vi "test Get Attribute as JSON.vi"(11 "Test Case In":refnum<class "Test Config From EXCEL.lvclass">) -> (0 "error out":errorcluster, 3 "Test Case Out":refnum<class "Test Config From EXCEL.lvclass">)   [LabVIEW 2020, in "Test Config From EXCEL.lvclass"]
uses:
  Test Config From EXCEL.lvclass
  Test Config From EXCEL.lvclass/Test Config From EXCEL.ctl
  <vilib>/JDP Science/JSONtext/JSONtext.lvlib
  <vilib>/Astemes/LUnit/Test Case.lvclass
  <vilib>/Peter/Open Xml/Source/Open Xml.lvlib
  Source/Config from EXCEL/Config from EXCEL.lvclass
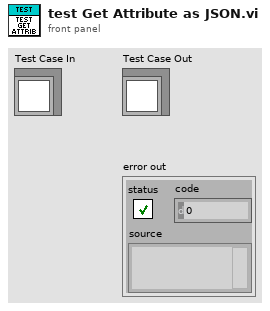
[diagram p1: front panel]
types:
  T1 = cluster{"Sheet Name":string, "Name":string, "Display Name":string, "Range or Cell Address":string}
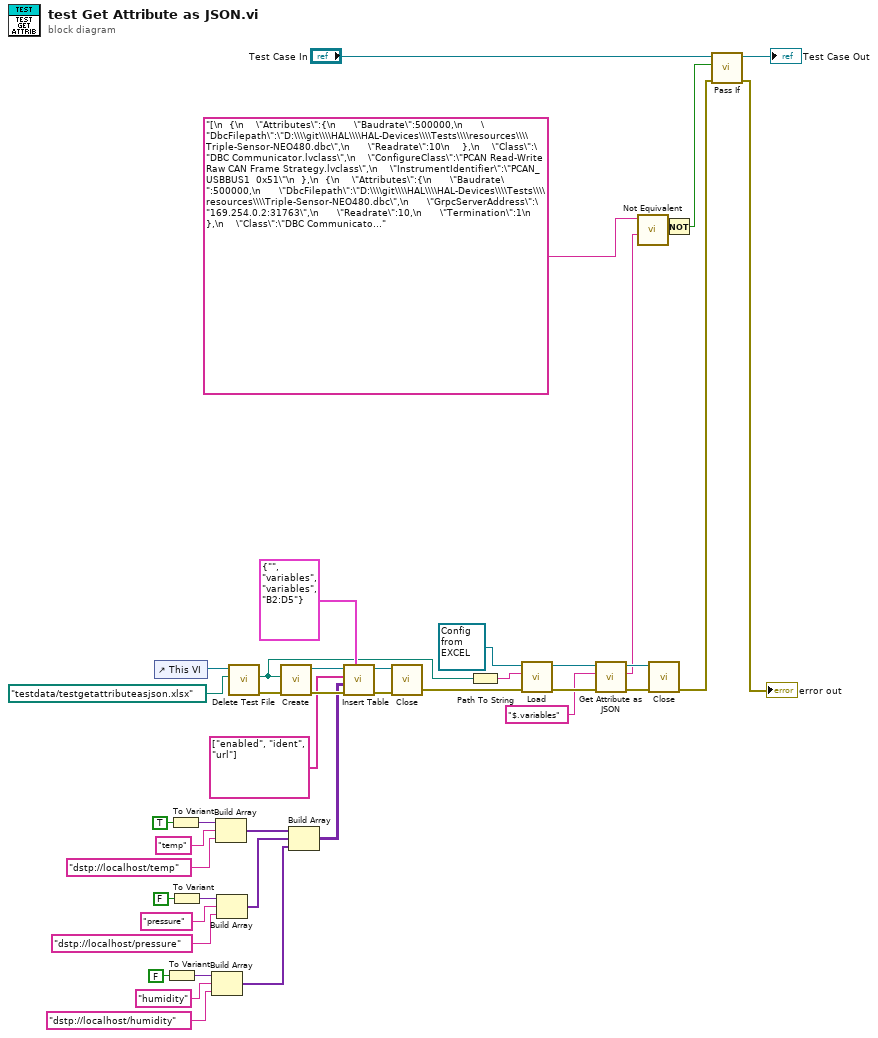
[diagram p0: block diagram]
diagram:
  n1 = control-ref of="This VI"() -> (w27:refnum<vi>)
  n2 = To Variant(anything=FALSE) -> (Variant=w11:variant)
  n3 = To Variant(anything=TRUE) -> (Variant=w20:variant)
  n4 = To Variant(anything=FALSE) -> (Variant=w14:variant)
  n5 = Build Array(w11, "humidity", "dstp://localhost/humidity") -> (w7:variant[])
  n6 = Build Array(w20, "temp", "dstp://localhost/temp") -> (w17:variant[])
  n7 = Build Array(w14, "pressure", "dstp://localhost/pressure") -> (w8:variant[])
  n8 = call "Delete Test File.vi"("name or relative path"=path "testdata/testgetattributeasjson.xlsx", "VI in"=w27) -> ("error out"=w25:errorcluster, "deleted path"=w4:path)  [unwired: 8 in]
  n9 = call <vilib>:"Create.vi"("error in"=w25, "Path"=w4) -> ("error out"=w24:errorcluster, "SpreadsheetDoc"=w5:refnum<k24>)  [unwired: 8 in]
  n10 = Build Array(w17, w8, w7) -> (w6:variant[][])
  n11 = call <vilib>:"Insert Table.vi"("Location"=T1 {"Sheet Name"="", "Name"="variables", "Display Name"="variables", "Range or Cell Address"="B2:D5"}, "error in"=w24, "Cell Values"=w6, "Header Names"=string[] ["enabled", "ident", "url"], "SpreadsheetDoc in"=w5) -> ("error out"=w3:errorcluster, "SpreadsheetDoc out"=w2:refnum<k24>)  [unwired: 5 in]
  n12 = call <vilib>:"Close.vi"("error in"=w3, "SpreadsheetDoc"=w2) -> ("error out"=w1:errorcluster)  [unwired: 9 in]
  n13 = Path To String(path=w4) -> (string=w38:string)
  n14 = call-dynamic "Load.vi"("error in"=w1, "Source"=w38, "Config from EXCEL in"=refnum<class "Config from EXCEL.lvclass"> refnum ("Configuration.lvlib:Config from EXCEL.lvclass")) -> ("error out"=w35:errorcluster, "Config from EXCEL out"=w36:refnum<class "Config from EXCEL.lvclass">)  [unwired: 7 in]
  n15 = call-dynamic "Get Attribute as JSON.vi"("error in"=w35, "Attribute"="$.variables", "Config from EXCEL in"=w36) -> ("error out"=w33:errorcluster, "<JSON>"=w29:string, "Config from EXCEL out"=w32:refnum<class "Config from EXCEL.lvclass">)  [unwired: 6 in]
  n16 = call <vilib>:"Not Equivalent.vi"("Other JSON"=w29, "JSON"="[\n  {\n    \"Attributes\":{\n      \"Baudrate\":500000,\n      \"DbcFilepath\":\"D:\\\\git\\\\HAL\\\\HAL-Devices\\\\Tests\\\\resources\\\\Triple-Sensor-NEO480.dbc\",\n      \"Readrate\":10\n    },\n    \"Class\":\"DBC Communicator.lvclass\",\n    \"ConfigureClass\":\"PCAN Read-Write Raw CAN Frame Strategy.lvclass\",\n    \"InstrumentIdentifier\":\"PCAN_USBBUS1  0x51\"\n  },\n  {\n    \"Attributes\":{\n      \"Baudrate\":500000,\n      \"DbcFilepath\":\"D:\\\\git\\\\HAL\\\\HAL-Devices\\\\Tests\\\\resources\\\\Triple-Sensor-NEO480.dbc\",\n      \"GrpcServerAddress\":\"169.254.0.2:31763\",\n      \"Readrate\":10,\n      \"Termination\":1\n    },\n    \"Class\":\"DBC Communicator.lvclass\",\n    \"ConfigureClass\":\"gRPC XNET Read Raw CAN Frame Strategy.lvclass\",\n    \"InstrumentIdentifier\":\"CAN1\"\n  },\n  {\n    \"Attributes\":{\n      \"Channels\":[\n        {\"CjcSource\":\"Constant Value\",\"CjcValue\":25,\"Enabled\":1,\"MaximumValue\":100,\"MinimumValue\":0,\"Name\":\"ai0\",\"ThermocoupleType\":\"J\",\"Units\":\"Deg C\"}\n      ],\n      \"Readrate\":10,\n      \"Timing\":{\n        \"ActiveEdge\":\"Rising\",\n        \"SampleClockSource\":\"OnboardClock\",\n        \"SampleMode\":\"Continuous Samples\",\n        \"SampleRate\":10,\n        \"SamplesPerChannel\":1000,\n        \"Type\":\"Sample Clock\"\n      },\n      \"Trigger\":{\"TriggerType\":\"No Trigger\"}\n    },\n    \"Class\":\"Thermometer Multichannel.lvclass\",\n    \"ConfigureClass\":\"DAQmx Thermocouple Continuous Read Strategy.lvclass\",\n    \"InstrumentIdentifier\":\"cDAQ9191-TC9210\"\n  }\n]") -> ("Not Equivalent"=w31:bool)  [unwired: 8 in]
  n17 = call-dynamic <vilib>:"Close.vi"("error in"=w33, "Config from EXCEL in"=w32) -> ("error out"=w37:errorcluster)  [unwired: 8 in, 1 out]
  n18 = Not(x=w31) -> (.not. x?=w30:bool)
  n19 = call <vilib>:"Pass If.vi"("error in (no error)"=w37, "Pass?"=w30, "LUnit Test Case In"="Test Case In") -> ("error out"=→"error out":errorcluster, "LUnit Test Case Out"=→"Test Case Out":refnum<class "Test Config From EXCEL.lvclass">)  [unwired: 7 in]
